vi "JigAndProductBarcodeScan.vi"(10 "Barcode":string, 11 "BarcodePosition":enum16{"JigBarcode", "ProductBarcode"}(ring)=enum."ProductBarcode") -> (2 "OK":bool, 3 "条码输出":string)   [LabVIEW 2014]
uses:
  axxon_Gold.vi
panel:
  out "治具条码扫描位":cluster{"X":dbl, "Y":dbl, "Z":dbl}
  in  "CleanAlarm":bool
  in  "Exit":bool
  in  "MenualScan":bool
  out "BarcodePosition":cluster{"X":dbl, "Y":dbl, "Z":dbl}
  out "NoPosition":cluster{"X":dbl, "Y":dbl, "Z":dbl}
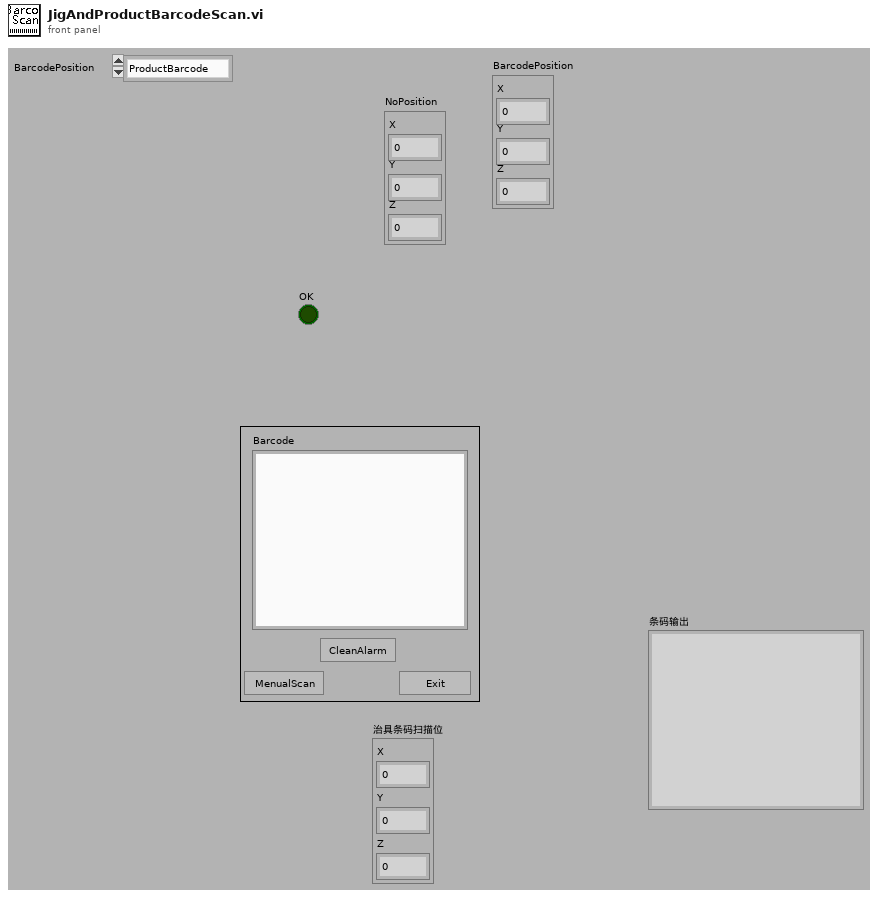
[diagram p1: front panel]
types:
  T1 = cluster{"Scan":bool, "NoPosition":cluster{"X":dbl, "Y":dbl, "Z":dbl}, "BarcodePosition":cluster{"X":dbl, "Y":dbl, "Z":dbl}}
  T2 = enum32{"Invalid", "Standard", "Closed", "Hidden", "Minimized", "Maximized"}
  T3 = cluster{"VISA resource name out":refnum<visa-resource-name>, "error out":errorcluster}
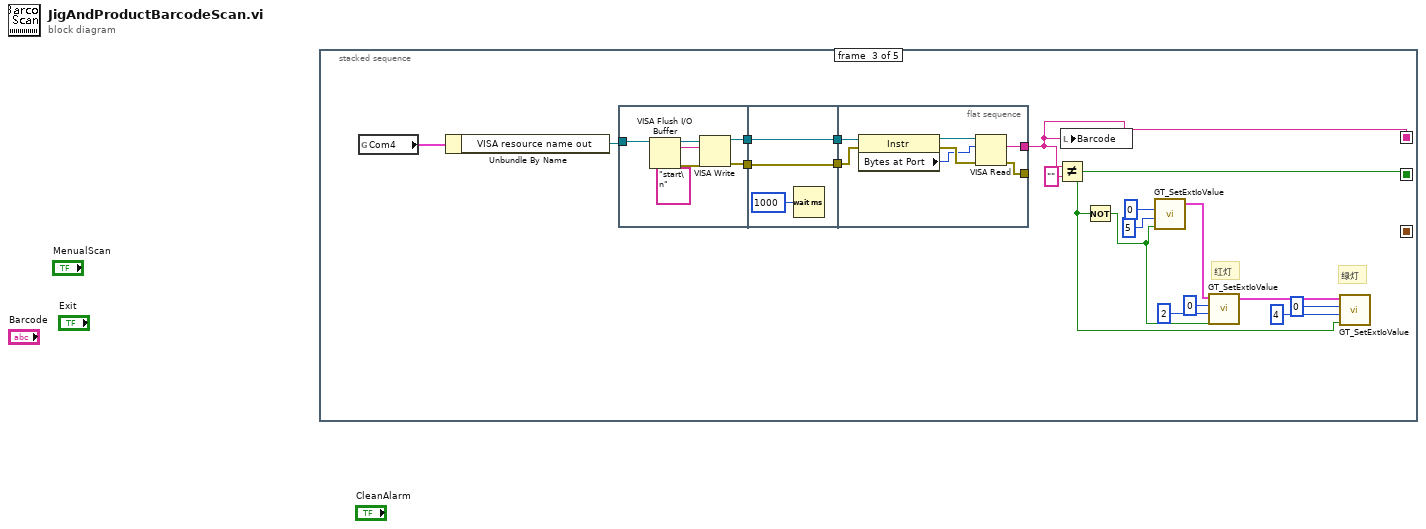
[diagram p0: block diagram]
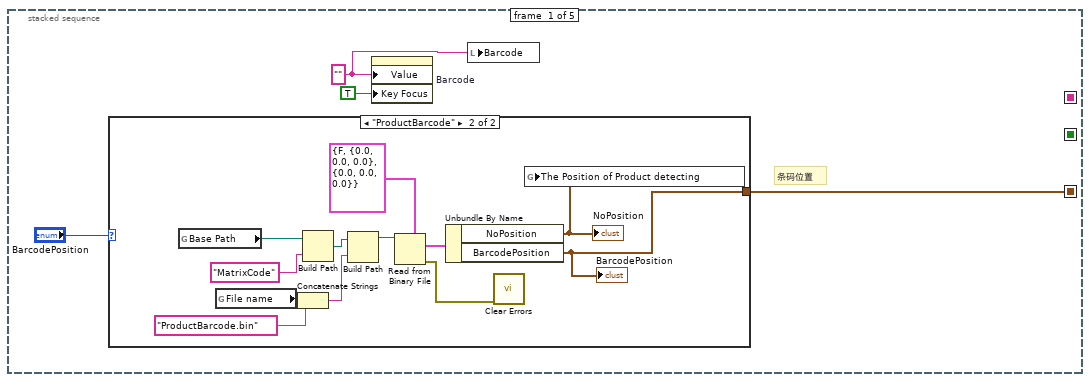
[diagram p2: hidden frame]
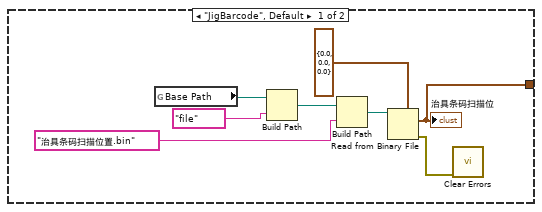
[diagram p3: hidden frame]
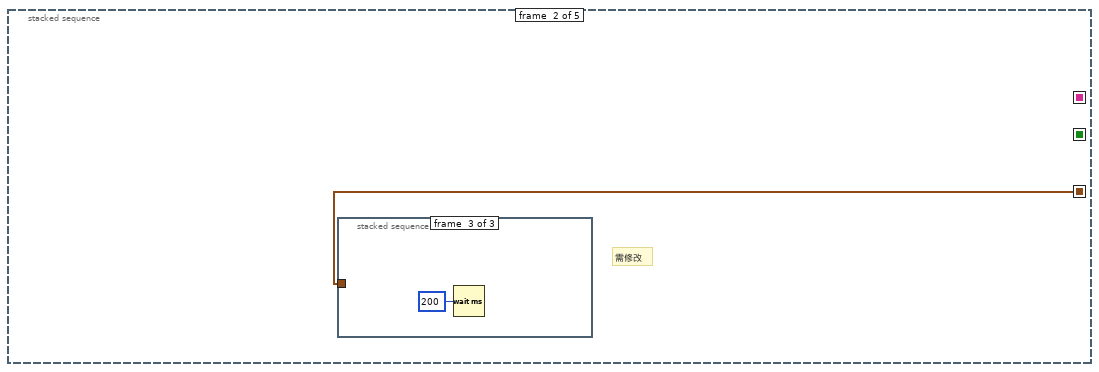
[diagram p4: hidden frame]
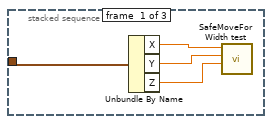
[diagram p5: hidden frame]
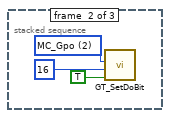
[diagram p6: hidden frame]
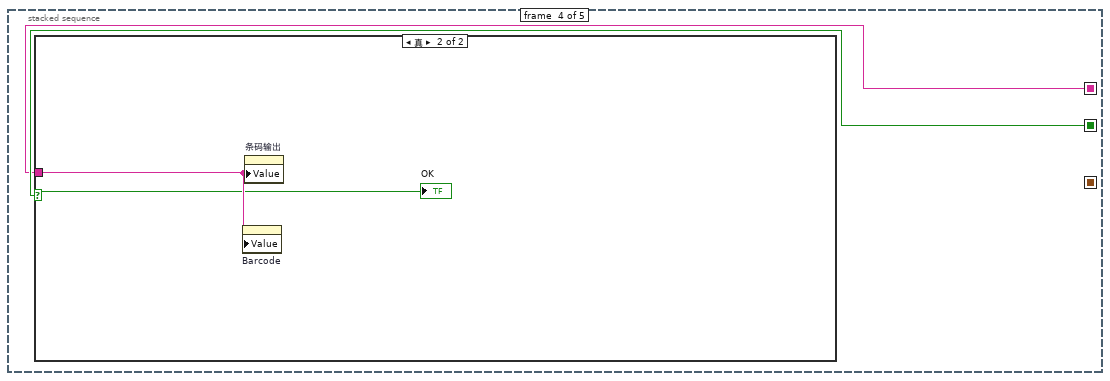
[diagram p7: hidden frame]
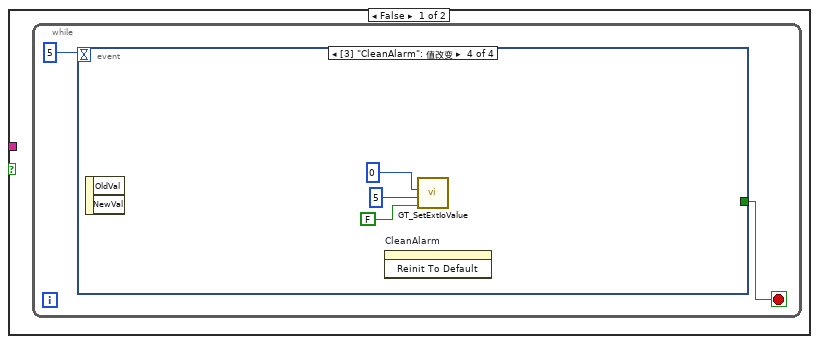
[diagram p8: hidden frame]
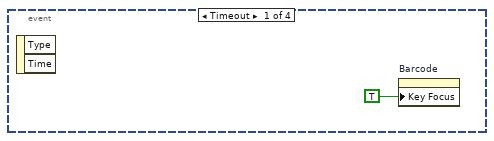
[diagram p9: hidden frame]
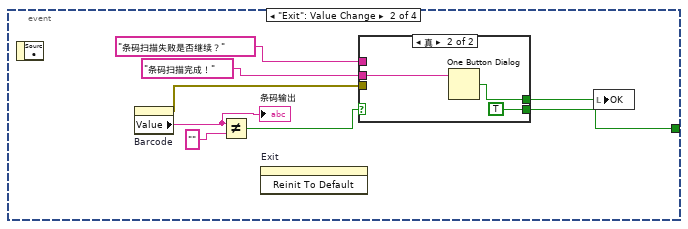
[diagram p10: hidden frame]
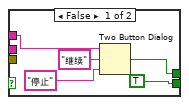
[diagram p11: hidden frame]
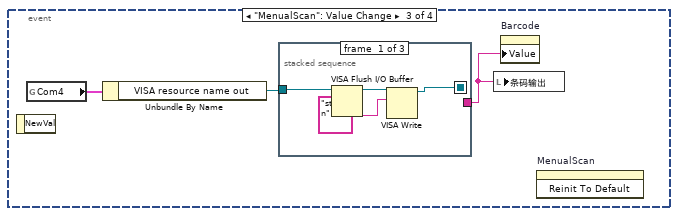
[diagram p12: hidden frame]
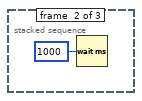
[diagram p13: hidden frame]
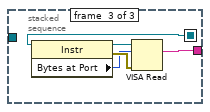
[diagram p14: hidden frame]
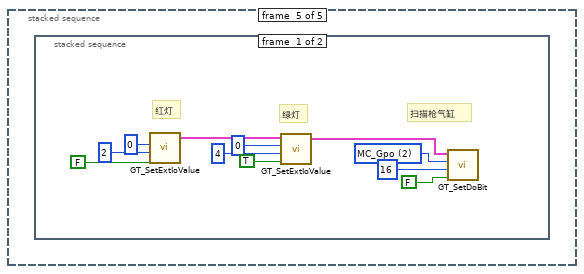
[diagram p15: hidden frame]
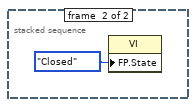
[diagram p16: hidden frame]
diagram:
  n1 = stacked-sequence {
    seq-local: [_ _ w34 _ _] -> [_ _ _ w69 _]
    seq-local: [_ _ w51 _ _] -> [_ _ _ w68 _]
    seq-local: [w1 _ _ _ _] -> [_ w25 _ _ _]
    frame #0 {
      w3 = "" ("条码")
      # "条码位置"
      n2 = case shown="\"ProductBarcode\"" "BarcodePosition" {
        tunnel: [w5 w13] -> w1
        frame "JigBarcode", Default {
          n3 = global read "axxon_Gold.vi" "Base Path"() -> (w12:path)
          n4 = Build Path(base path=w12, name or relative path="file" ("名称或相对路径")) -> (appended path=w10:path)
          n5 = Build Path(base path=w10, name or relative path="治具条码扫描位置.bin" ("名称或相对路径")) -> (appended path=w8:path)
          n6 = Read from Binary File(5:cluster{"X":dbl, "Y":dbl, "Z":dbl} {"X"=0.0, "Y"=0.0, "Z"=0.0} ("治具条码扫描位置"), 11:w8) -> (0:w7:errorcluster, 2:w5:cluster{"X":dbl, "Y":dbl, "Z":dbl})  [unwired: 4 in, 2 out]
          "治具条码扫描位" <- w5
          n7 = call <vilib>:"Clear Errors.vi"("error in (no error)"=w7) -> ()  [unwired: 5 in, 2 out]
        }
        frame "ProductBarcode" {
          n8 = global read "axxon_Gold.vi" "Base Path"() -> (w23:path)
          n9 = global read "axxon_Gold.vi" "File name"() -> (w21:string)
          n10 = Concatenate Strings(w21, "ProductBarcode.bin" ("字符串")) -> (w20:string)
          n11 = Build Path(base path=w23, name or relative path="MatrixCode" ("名称或相对路径")) -> (appended path=w22:path)
          n12 = Build Path(base path=w22, name or relative path=w20) -> (appended path=w19:path)
          n13 = Read from Binary File(5:T1 {"Scan"=FALSE, "NoPosition"={"X"=0.0, "Y"=0.0, "Z"=0.0}, "BarcodePosition"={"X"=0.0, "Y"=0.0, "Z"=0.0}}, 11:w19) -> (0:w14:errorcluster, 2:w17:T1)  [unwired: 4 in, 2 out]
          n14 = Unbundle By Name(w17) -> ("NoPosition"=w16:cluster{"X":dbl, "Y":dbl, "Z":dbl}, "BarcodePosition"=w13:cluster{"X":dbl, "Y":dbl, "Z":dbl})
          "NoPosition" <- w16
          "BarcodePosition" <- w13
          n15 = call <vilib>:"Clear Errors.vi"("error in (no error)"=w14) -> ()  [unwired: 5 in, 2 out]
          n16 = global write "axxon_Gold.vi" "The Position of Product detecting"(w16) -> ()
        }
      }
      n17 = property on="Barcode" class="Str"("Value"=w3, "Key Focus"=TRUE ("键选中")) -> ()  [unwired: 2 in, 2 out]
      n18 = local write "Barcode"(w3) -> ()
    }
    frame #1 {
      # "需修改"
      n19 = stacked-sequence {
        tunnel: w25 -> [w26 _ _]
        frame #0 {
          n20 = Unbundle By Name(w26) -> ("X"=w29:dbl, "Y"=w28:dbl, "Z"=w27:dbl)
          n21 = call "SafeMoveFor Width test.vi"("Z"=w27, "Y"=w28, "X"=w29) -> ()  [unwired: 8 in, 1 out]
        }
        frame #1 {
          w30 = i16 2 items=["MC_Enable", "MC_Clear", "MC_Gpo"] ("doType")
          n22 = call "GT_SetDoBit.vi"("Value"=TRUE, "doIndex"=i16 16, "doType"=w30) -> ()  [unwired: 8 in, 1 out]
        }
        frame #2 {
          n23 = Wait (ms)(milliseconds to wait=u32 200 ("等待时间（毫秒）")) -> ()  [unwired: 1 out]
        }
      }
    }
    frame #2 {
      # "绿灯"
      # "红灯"
      n24 = global read "axxon_Gold.vi" "Com4"() -> (w46:T3)
      n25 = Unbundle By Name(w46) -> ("VISA resource name out"=w45:refnum<visa-resource-name>)
      n26 = flat-sequence {
        tunnel: w45 -> [w57]
        tunnel: [w55] -> w50
        tunnel: [w54] -> w49
        tunnel: w50 -> [w59]
        tunnel: [w59] -> w48
        tunnel: w49 -> [w58]
        tunnel: [w58] -> w47
        tunnel: w48 -> [w67]
        tunnel: w47 -> [w66]
        tunnel: [w62] -> _
        tunnel: [w61] -> w51
        frame #0 {
          n27 = VISA Flush I/O Buffer(VISA resource name=w57) -> (VISA resource name out=w53:refnum<visa-resource-name>, error out=w52:errorcluster)  [unwired: 2 in]
          n28 = VISA Write(VISA resource name=w53, write buffer="start\n" ("写入缓冲区"), error in (no error)=w52) -> (VISA resource name out=w54:refnum<visa-resource-name>, error out=w55:errorcluster)  [unwired: 1 out]
        }
        frame #1 {
          n29 = Wait (ms)(milliseconds to wait=u32 1000 ("等待时间（毫秒）")) -> ()  [unwired: 1 out]
        }
        frame #2 {
          n30 = property class="Instr"(reference=w66, error in=w67) -> (reference out=w65:refnum<visa-resource-name>, error out=w64:errorcluster, "Bytes at Port"=w63:u32)
          n31 = VISA Read(VISA resource name=w65, byte count=w63, error in (no error)=w64) -> (read buffer=w61:string, error out=w62:errorcluster)  [unwired: 2 out]
        }
      }
      n32 = Not Equal?(x=w51, y="") -> (x != y?=w34:bool)
      n33 = local write "Barcode"(w51) -> ()
      n34 = Not(x=w34) -> (.not. x?=w35:bool)
      n35 = call "GT_SetExtIoValue.vi"("Value"=w35, "index"=5, "mdl"=0) -> ("rtn_Out"=w36:cluster{"rtn":i16, "Func":string})  [unwired: 3 in]
      n36 = call "GT_SetExtIoValue.vi"("Value"=w35, "index"=2, "mdl"=0, "rtn_In"=w36) -> ("rtn_Out"=w39:cluster{"rtn":i16, "Func":string})  [unwired: 2 in]
      n37 = call "GT_SetExtIoValue.vi"("Value"=w34, "index"=4, "mdl"=0, "rtn_In"=w39) -> ()  [unwired: 2 in, 1 out]
    }
    frame #3 {
      n38 = case shown="真" w69 {
        selector: w69 -> [_ w105]
        tunnel: w68 -> [_ w106]
        frame False {
          n39 = while {
            stop <- w70 stop-if-true
            n40 = event shown="[3] \"CleanAlarm\": 值改变" {
              selector: _ -> [_ _ _ _]
              dyn-events: _ -> [_ _ _ _]
              timeout: 5 -> [_ _ _ _]
              tunnel: [_ w73 _ _] -> w70
              event Timeout {
                n41 = event-data() -> ()  [unwired: 1 in, 2 out]
                n42 = property on="Barcode" class="Str"("Key Focus"=TRUE ("键选中")) -> ()  [unwired: 2 in, 2 out]
              }
              event "Exit": Value Change {
                n43 = event-data() -> ()  [unwired: 1 in, 1 out]
                n44 = property on="Barcode" class="Str"() -> (error out=w78:errorcluster, "Value"=w79:string)  [unwired: 2 in, 1 out]
                "条码输出" <- w79
                n45 = Not Equal?(x=w79, y="") -> (x != y?=w74:bool)
                n46 = invoke on="Exit" class="Bool" method="Reinit To Default"() -> ()  [unwired: 3 in, 3 out]
                n47 = case shown="真" w74 {
                  tunnel: w78 -> [_ _]
                  tunnel: "条码扫描失败是否继续？" ("消息") -> [w85 _]
                  tunnel: [w82 w87] -> w76
                  tunnel: "条码扫描完成！" ("消息") -> [_ w88]
                  tunnel: [TRUE TRUE] -> w73
                  frame False {
                    n48 = Two Button Dialog(message=w85, 1:"停止" ("F按钮名称（“取消”）"), 2:"继续" ("T按钮名称（“确定”）")) -> (T button?=w82:bool)
                  }
                  frame True {
                    n49 = One Button Dialog(message=w88) -> (true=w87:bool)  [unwired: 1 in]
                  }
                }
                n50 = local write "OK"(w76) -> ()
              }
              event "MenualScan": Value Change {
                n51 = event-data() -> ()  [unwired: 1 in, 1 out]
                n52 = global read "axxon_Gold.vi" "Com4"() -> (w91:T3)
                n53 = Unbundle By Name(w91) -> ("VISA resource name out"=w90:refnum<visa-resource-name>)
                n54 = stacked-sequence {
                  seq-local: [w93 _ _] -> [_ _ w97]
                  tunnel: w90 -> [w95 _ _]
                  tunnel: [_ _ w98] -> w89
                  frame #0 {
                    n55 = VISA Flush I/O Buffer(VISA resource name=w95) -> (VISA resource name out=w92:refnum<visa-resource-name>)  [unwired: 2 in, 1 out]
                    n56 = VISA Write(VISA resource name=w92, write buffer="start\n" ("写入缓冲区")) -> (VISA resource name out=w93:refnum<visa-resource-name>)  [unwired: 1 in, 2 out]
                  }
                  frame #1 {
                    n57 = Wait (ms)(milliseconds to wait=u32 1000 ("等待时间（毫秒）")) -> ()  [unwired: 1 out]
                  }
                  frame #2 {
                    n58 = property class="Instr"(reference=w97) -> (reference out=w101:refnum<visa-resource-name>, error out=w100:errorcluster, "Bytes at Port"=w99:u32)  [unwired: 1 in]
                    n59 = VISA Read(VISA resource name=w101, byte count=w99, error in (no error)=w100) -> (read buffer=w98:string)  [unwired: 3 out]
                  }
                }
                n60 = local write "条码输出"(w89) -> ()
                n61 = property on="Barcode" class="Str"("Value"=w89) -> ()  [unwired: 2 in, 2 out]
                n62 = invoke on="MenualScan" class="Bool" method="Reinit To Default"() -> ()  [unwired: 3 in, 3 out]
              }
              event "CleanAlarm": Value Change {
                n63 = event-data() -> ()  [unwired: 1 in, 2 out]
                n64 = invoke on="CleanAlarm" class="Bool" method="Reinit To Default"() -> ()  [unwired: 3 in, 3 out]
                n65 = call "GT_SetExtIoValue.vi"("Value"=FALSE, "index"=5, "mdl"=0) -> ()  [unwired: 3 in, 1 out]
              }
            }
          }
        }
        frame True {
          n66 = property on="Barcode" class="Str"("Value"=w106) -> ()  [unwired: 2 in, 2 out]
          n67 = property on="条码输出" class="Str"("Value"=w106) -> ()  [unwired: 2 in, 2 out]
          "OK" <- w105
        }
      }
    }
    frame #4 {
      n68 = stacked-sequence {
        frame #0 {
          w115 = i16 2 items=["MC_Enable", "MC_Clear", "MC_Gpo"] ("doType")
          # "扫描枪气缸"
          # "绿灯"
          # "红灯"
          n69 = call "GT_SetExtIoValue.vi"("Value"=FALSE, "index"=2, "mdl"=0) -> ("rtn_Out"=w111:cluster{"rtn":i16, "Func":string})  [unwired: 3 in]
          n70 = call "GT_SetExtIoValue.vi"("Value"=TRUE, "index"=4, "mdl"=0, "rtn_In"=w111) -> ("rtn_Out"=w107:cluster{"rtn":i16, "Func":string})  [unwired: 2 in]
          n71 = call "GT_SetDoBit.vi"("Value"=FALSE, "doIndex"=i16 16, "doType"=w115, "rtn_In"=w107) -> ()  [unwired: 7 in, 1 out]
        }
        frame #1 {
          n72 = property class="VI"("FP.State"=T2."Closed" ("前面板窗口:状态")) -> ()  [unwired: 2 in, 2 out]
        }
      }
    }
  }
